vi "Calculate Driving Direction of Tank2.vi"(8 "error in (no error)":errorcluster, 10 "obstacle angles (rad)":dbl[](array[numeric]), 11 "obstacle distances (m)":dbl[](array[numeric])) -> (0 "error out":errorcluster, 3 "steering frame velocity":dbl[](array[numeric]))   [LabVIEW 2012]
doc: "Calculates the velocity vector of the robot required to avoid obstacles, based on the scanned data."
uses:
  <vilib>/robotics/Obstacle Avoidance/Simple Vector Field Histogram/Panic Range.ctl
  <vilib>/Utility/AngleManip/Degrees to Radians (Scalar DBL).vi
  <vilib>/robotics/Obstacle Avoidance/Simple Vector Field Histogram/NI_Robotics_Simple Vector Field Histogram.lvlib
  <vilib>/Utility/AngleManip/NI_AngleManipulation.lvlib
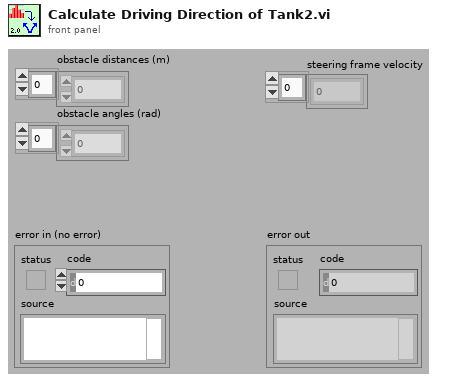
[diagram p1: front panel]
types:
  T1 = typedef "NI_Robotics_Simple Vector Field Histogram.lvlib/Panic Range.ctl" = cluster{"panic threshold distance (0)":dbl, "panic threshold angle (0)":dbl}
  T2 = typedef "NI_Robotics_Simple Vector Field Histogram.lvlib/Obstacle Description.ctl" = cluster{"angle to obstacle":dbl, "distance to obstacle":dbl}
  T3 = typedef "NI_Robotics_Simple Vector Field Histogram.lvlib/Gap Description.ctl" = cluster{"angle to gap":dbl, "size of gap":dbl}
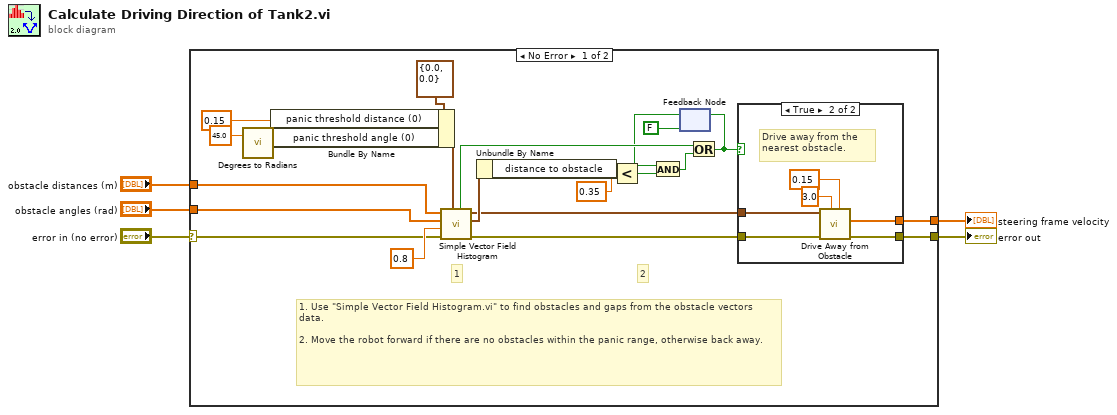
[diagram p0: block diagram]
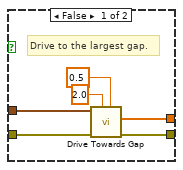
[diagram p2: hidden frame]
diagram:
  n1 = case shown="No Error" "error in (no error)" {
    selector: "error in (no error)" -> [w10 w40]
    tunnel: [w11 w40] -> w5
    tunnel: "obstacle distances (m)" -> [w9 _]
    tunnel: "obstacle angles (rad)" -> [w8 _]
    tunnel: [w7 _] -> w1
    frame No Error {
      # "2"
      # "1"
      # "1. Use \"Simple Vector Field Histogram.vi\" to find obstacles and gaps from the obstacle vectors data.\n\n2. Move the robot forward if there are no obstacles within the panic range, otherwise back away."
      n2 = call-poly <vilib>:"Degrees to Radians.vi"("angle (deg)"=45.0 ("panic threshold angle (rad)")) -> ("angle (rad)"=w27:dbl)  [unwired: 2 in]
      n3 = Bundle By Name(cluster=T1 {"panic threshold distance (0)"=0.0, "panic threshold angle (0)"=0.0} ("panic range"), "panic threshold distance (0)"=0.15 ("panic threshold distance (m)"), "panic threshold angle (0)"=w27) -> (w15:T1)
      n4 = call <vilib>:"Simple Vector Field Histogram.vi"("panic range"=w15, "error in (no error)"=w10, "distance threshold"=0.8 ("distance threshold (m)"), "direction angles"=w8, "distances"=w9) -> ("error out"=w12:errorcluster, "nearest obstacle"=w17:T2, "largest gap"=w6:T3, "obstacle within panic range"=w22:bool)  [unwired: 2 in, 1 out]
      n5 = Unbundle By Name(w17) -> ("distance to obstacle"=w18:dbl)
      n6 = Less?(x=w18, y=0.35) -> (x < y?=w20:bool)
      n7 = feedback #1(FALSE ("obstacle within panic range")) -> (w21:bool)
      n8 = And(x=w21, y=w20) -> (x .and. y?=w23:bool)
      n9 = Or(x=w22, y=w23) -> (x .or. y?=w25:bool)
      n10 = feedback-in #1(w25) -> ()
      n11 = case shown="True" w25 {
        tunnel: w6 -> [w32 w37]
        tunnel: w12 -> [w33 w39]
        tunnel: [w31 w38] -> w11
        tunnel: [w30 w36] -> w7
        frame False {
          # "Drive to the largest gap."
          n12 = call "Drive Towards Gap.vi"("max forward velocity (m/s)"=0.5, "max angular velocity (rad/s)"=2.0, "error in (no error)"=w33, "gap"=w32) -> ("error out"=w31:errorcluster, "steering frame velocity"=w30:dbl[])  [unwired: 6 in]
        }
        frame True {
          # "Drive away from the nearest obstacle."
          n13 = call "Drive Away from Obstacle.vi"("max reverse velocity (m/s)"=0.15, "max angular velocity (rad/s)"=3.0, "error in (no error)"=w39, "gap"=w37) -> ("error out"=w38:errorcluster, "steering frame velocity"=w36:dbl[])  [unwired: 6 in]
        }
      }
    }
    frame Error {
    }
  }
  "error out" <- w5
  "steering frame velocity" <- w1
